vi "Destroy Request Events.vi"(8 "error in":errorcluster) -> (0 "error out":errorcluster)   [LabVIEW 2025, in "Scripting Server.lvlib"]
doc: "Destroy the requests user events, even if there is an incoming error.\n\n<b>NOTE</b>: The contents of this VI are automatically generated and modified by the <b>Tools > DQMH Consortium > DQMH</b> utilities. Consider using those utilities instead of making your own modifications to this VI.\n_____\nBased on DQMH Dev Tools: Project Template 7.1.0.1503."
uses:
  Scripting Server.lvlib
panel:
  # "NOTE: The contents of this VI are automatically generated and modified by the Tools > DQMH Consortium > DQMH utilities. Consider using those utilities instead of making your own modifications to this VI."
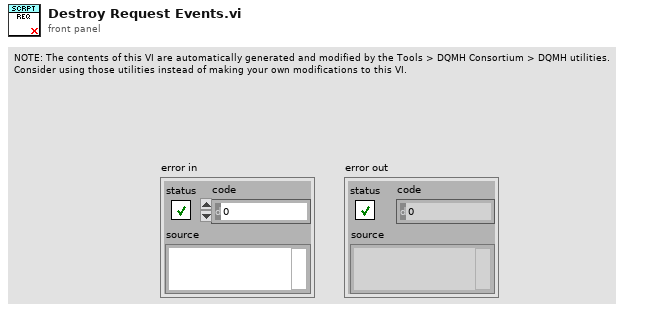
[diagram p1: front panel]
types:
  T1 = typedef "Scripting Server.lvlib/Request Events--cluster.ctl" = cluster{"Stop Module":refnum<user-event>, "Show Panel":refnum<user-event>, "Hide Panel":refnum<user-event>, "Get Module Execution Status":refnum<user-event>, "Show Diagram":refnum<user-event>, "New VI":refnum<user-event>, "Add Object":refnum<user-event>, "Connect Objects":refnum<user-event>, "Get Object Terminals":refnum<user-event>, "get vi error list":refnum<user-event>, "Cleanup VI":refnum<user-event>, "create_control":refnum<user-event>, "Run VI":refnum<user-event>, "add_to_selection":refnum<user-event>, "clear_selection_list":refnum<user-event>, "remove_from_selection":refnum<user-event>, "enclose_selection":refnum<user-event>}
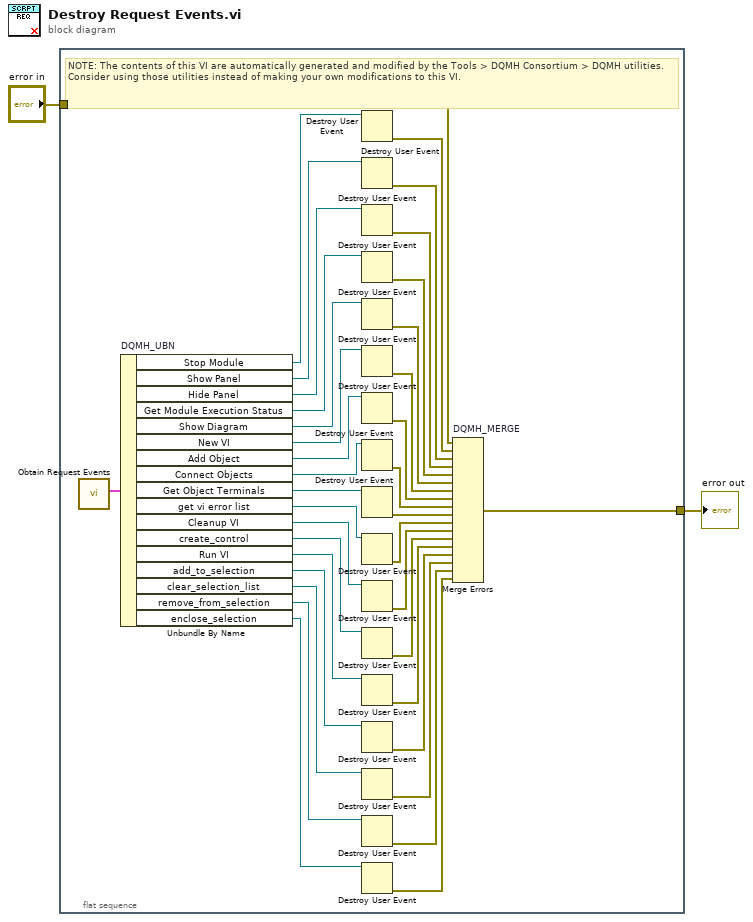
[diagram p0: block diagram]
diagram:
  n1 = flat-sequence {
    tunnel: [w38] -> w2
    tunnel: "error in" -> [w31]
    frame #0 {
      # "NOTE: The contents of this VI are automatically generated and modified by the Tools > DQMH Consortium > DQMH utilities. Consider using those utilities instead of making your own modifications to this VI."
      n2 = call "Obtain Request Events.vi"() -> ("Scripting Server Request Events"=w37:T1)  [unwired: 10 in, 1 out]
      n3 = Unbundle By Name "DQMH_UBN"(w37) -> ("Stop Module"=w36:refnum<user-event>, "Show Panel"=w33:refnum<user-event>, "Hide Panel"=w32:refnum<user-event>, "Get Module Execution Status"=w29:refnum<user-event>, "Show Diagram"=w27:refnum<user-event>, "New VI"=w25:refnum<user-event>, "Add Object"=w23:refnum<user-event>, "Connect Objects"=w21:refnum<user-event>, "Get Object Terminals"=w19:refnum<user-event>, "get vi error list"=w17:refnum<user-event>, "Cleanup VI"=w15:refnum<user-event>, "create_control"=w13:refnum<user-event>, "Run VI"=w11:refnum<user-event>, "add_to_selection"=w9:refnum<user-event>, "clear_selection_list"=w7:refnum<user-event>, "remove_from_selection"=w5:refnum<user-event>, "enclose_selection"=w3:refnum<user-event>)
      n4 = Destroy User Event(user event=w36) -> (error out=w39:errorcluster)  [unwired: 1 in]
      n5 = Destroy User Event(user event=w33) -> (error out=w35:errorcluster)  [unwired: 1 in]
      n6 = Destroy User Event(user event=w32) -> (error out=w34:errorcluster)  [unwired: 1 in]
      n7 = Destroy User Event(user event=w29) -> (error out=w30:errorcluster)  [unwired: 1 in]
      n8 = Destroy User Event(user event=w27) -> (error out=w28:errorcluster)  [unwired: 1 in]
      n9 = Destroy User Event(user event=w25) -> (error out=w26:errorcluster)  [unwired: 1 in]
      n10 = Destroy User Event(user event=w23) -> (error out=w24:errorcluster)  [unwired: 1 in]
      n11 = Destroy User Event(user event=w21) -> (error out=w22:errorcluster)  [unwired: 1 in]
      n12 = Destroy User Event(user event=w19) -> (error out=w20:errorcluster)  [unwired: 1 in]
      n13 = Destroy User Event(user event=w17) -> (error out=w18:errorcluster)  [unwired: 1 in]
      n14 = Destroy User Event(user event=w15) -> (error out=w16:errorcluster)  [unwired: 1 in]
      n15 = Destroy User Event(user event=w13) -> (error out=w14:errorcluster)  [unwired: 1 in]
      n16 = Destroy User Event(user event=w11) -> (error out=w12:errorcluster)  [unwired: 1 in]
      n17 = Destroy User Event(user event=w9) -> (error out=w10:errorcluster)  [unwired: 1 in]
      n18 = Destroy User Event(user event=w7) -> (error out=w8:errorcluster)  [unwired: 1 in]
      n19 = Destroy User Event(user event=w5) -> (error out=w6:errorcluster)  [unwired: 1 in]
      n20 = Destroy User Event(user event=w3) -> (error out=w4:errorcluster)  [unwired: 1 in]
      n21 = Merge Errors "DQMH_MERGE"(w31, w39, w35, w34, w30, w28, w26, w24, w22, w20, w18, w16, w14, w12, w10, w8, w6, w4) -> (w38:errorcluster)
    }
  }
  "error out" <- w2
